vi "RTS Close TDMS.vi"(7 "RTS Config Setup Input":T2, 8 "Error In":errorcluster, 10 "Tree Selection":T1, 11 "TDMS Data Save in":T11) -> (0 "Error Out":errorcluster, 3 "RTS Config Setup Output":T2)   [LabVIEW 2016]
uses:
  Type Definitions/RTS TDMS Filename Locations.ctl
  Type Definitions/RTS Wago Config.ctl
  Type Definitions/RTS APLUS Config.ctl
  Type Definitions/RTS Yokogawa MX Config.ctl
  Type Definitions/RTS Replay Server Control.ctl
  Type Definitions/RTS Server Configuration.ctl
  Type Definitions/RTS Configuration Setup.ctl
  Type Definitions/RTS Station Settions TCP Comms.ctl
  Type Definitions/RTS Chamber Save Status.ctl
  Type Definitions/RTS Room Selector.ctl
  Type Definitions/RTS Test Pattern.ctl
  Type Definitions/RTS Save References.ctl
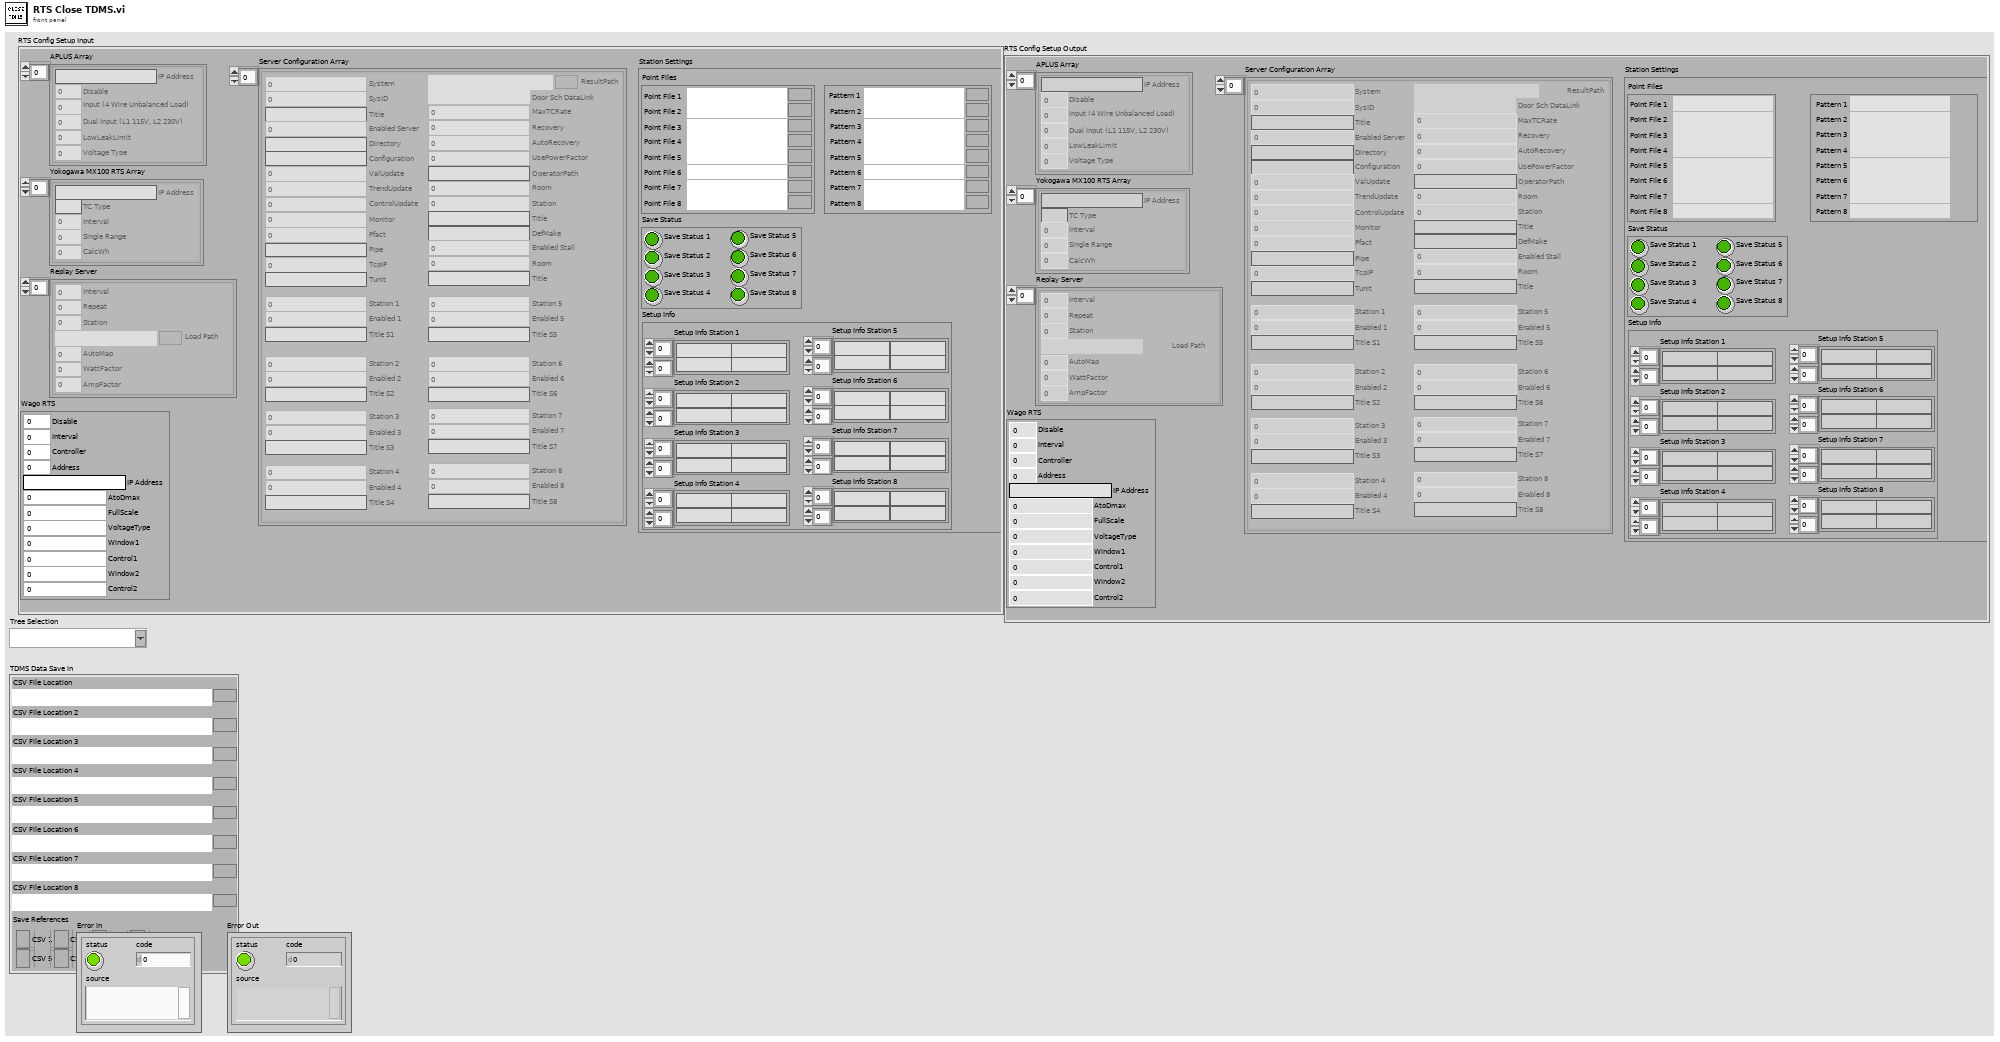
[diagram p1: front panel]
types:
  T1 = typedef "RTS Room Selector.ctl" = string
  T2 = typedef "RTS Configuration Setup.ctl" = cluster{"Wago RTS":T3, "APLUS Array":T4[], "Yokogawa MX100 RTS Array":T5[], "Replay Server":T6[], "Server Configuration Array":T7[], "Station Settings":T8}
  T3 = typedef "RTS Wago Config.ctl" = cluster{"Disable":u16, "Interval":u16, "Controller":u16, "Address":u16, "IP Address":string, "AtoDmax":u16, "FullScale":u16, "VoltageType":u16, "Window1":u16, "Control1":u16, "Window2":u16, "Control2":u16}
  T4 = typedef "RTS APLUS Config.ctl" = cluster{"Disable":u16, "IP Address":string, "Input (4 Wire Unbalanced Load)":u16, "Dual Input (L1 115V, L2 230V)":u16, "LowLeakLimit":dbl, "Voltage Type":u16}
  T5 = typedef "RTS Yokogawa MX Config.ctl" = cluster{"IP Address":string, "TC Type":string, "Interval":u16, "Single Range":u16, "CalcWh":u16}
  T6 = typedef "RTS Replay Server Control.ctl" = cluster{"Interval":i16, "Repeat":u16, "Station":u16, "Load Path":path, "AutoMap":u16, "WattFactor":dbl, "AmpFactor":dbl}
  T7 = typedef "RTS Server Configuration.ctl" = cluster{"System":u16, "SysID":u16, "Title":string, "Enabled Server":u16, "Directory":string, "Configuration":string, "ValUpdate":u16, "TrendUpdate":u16, "ControlUpdate":u16, "Monitor":u16, "Pfact":u16, "Pipe":string, "TcpIP":u16, "Tunit":string, "ResultPath":path, "Door Sch DataLink":path, "MaxTCRate":u16, "Recovery":u16, "AutoRecovery":u16, "UsePowerFactor":u16, "OperatorPath":string, "Room":u16, "Station":u16, "Title":string, "DefMake":string, "Enabled Stall":u16, "Room":u16, "Title":string, "Station 1":u16, "Enabled 1":u16, "Station 2":u16, "Enabled 2":u16, "Station 3":u16, "Enabled 3":u16, "Station 4":u16, "Enabled 4":u16, "Station 5":u16, "Enabled 5":u16, "Station 6":u16, "Enabled 6":u16, "Station 7":u16, "Enabled 7":u16, "Station 8":u16, "Enabled 8":u16, "Title S1":string, "Title S2":string, "Title S3":string, "Title S5":string, "Title S6":string, "Title S7":string, "Title S8":string, "Title S4":string}
  T8 = typedef "RTS Station Settions TCP Comms.ctl" = cluster{"Point Files":cluster{"Point File 1":path, "Point File 2":path, "Point File 3":path, "Point File 4":path, "Point File 5":path, "Point File 6":path, "Point File 7":path, "Point File 8":path}, "Save Status":T9, "Setup Info":cluster{"Setup Info Station 1":string[][], "Setup Info Station 2":string[][], "Setup Info Station 3":string[][], "Setup Info Station 4":string[][], "Setup Info Station 5":string[][], "Setup Info Station 6":string[][], "Setup Info Station 7":string[][], "Setup Info Station 8":string[][]}, "Chamber Test Pattern":T10}
  T9 = typedef "RTS Chamber Save Status.ctl" = cluster{"Save Status 1":bool, "Save Status 2":bool, "Save Status 3":bool, "Save Status 4":bool, "Save Status 5":bool, "Save Status 6":bool, "Save Status 7":bool, "Save Status 8":bool}
  T10 = typedef "RTS Test Pattern.ctl" = cluster{" Pattern 1":path, "Pattern 2":path, "Pattern 3":path, "Pattern 4":path, "Pattern 5":path, "Pattern 6":path, "Pattern 7":path, "Pattern 8":path}
  T11 = typedef "RTS TDMS Filename Locations.ctl" = cluster{"CSV File Location":path, "CSV File Location 2":path, "CSV File Location 3":path, "CSV File Location 4":path, "CSV File Location 5":path, "CSV File Location 6":path, "CSV File Location 7":path, "CSV File Location 8":path, "Save References":T12}
  T12 = typedef "RTS Save References.ctl" = cluster{"CSV 1":refnum<file>, "CSV 2":refnum<file>, "CSV 3":refnum<file>, "CSV 4":refnum<file>, "CSV 5":refnum<file>, "CSV 6":refnum<file>, "CSV 7":refnum<file>, "CSV 8":refnum<file>}
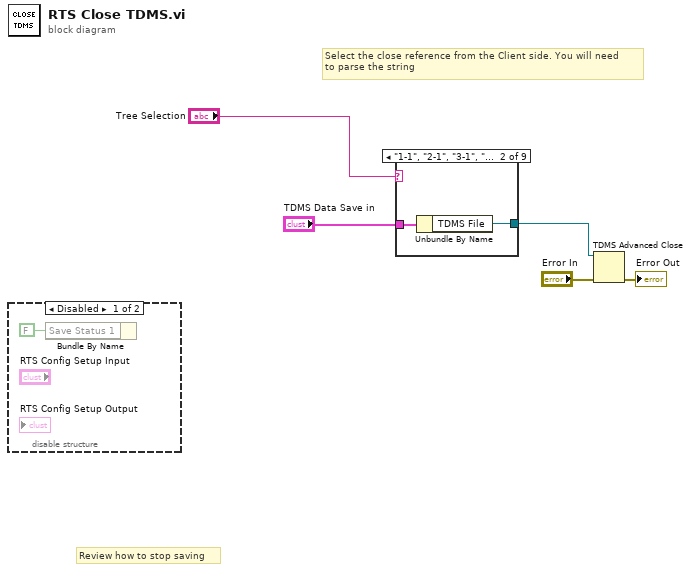
[diagram p0: block diagram]
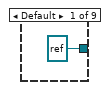
[diagram p3: hidden frame]
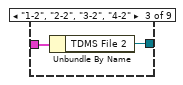
[diagram p4: hidden frame]
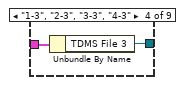
[diagram p5: hidden frame]
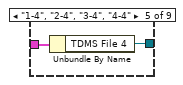
[diagram p6: hidden frame]
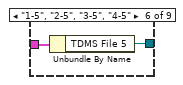
[diagram p7: hidden frame]
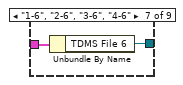
[diagram p8: hidden frame]
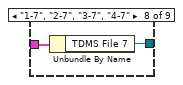
[diagram p9: hidden frame]
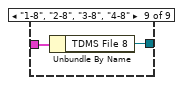
[diagram p10: hidden frame]
diagram:
  # "Review how to stop saving"
  # "Select the close reference from the Client side. You will need\nto parse the string"
  n1 = disable-structure shown="Disabled" {
    frame Disabled {
      n2 = Bundle By Name("Save Status 1"=FALSE ("Station Saving 8")) -> ()  [unwired: 1 in, 1 out]
    }
    frame Enabled {
    }
  }
  n3 = case shown="\"1-1\", \"2-1\", \"3-1\", \"4-1\"" "Tree Selection" {
    tunnel: "TDMS Data Save in" -> [_ w9 w11 w13 w15 w17 w19 w21 w23]
    tunnel: [refnum<k34> refnum ("TDMS File 8") w8 w10 w12 w14 w16 w18 w20 w22] -> w2
    frame Default {
    }
    frame "1-1", "2-1", "3-1", "4-1" {
      n4 = Unbundle By Name(w9) -> ("TDMS File"=w8:refnum<k34>)
    }
    frame "1-2", "2-2", "3-2", "4-2" {
      n5 = Unbundle By Name(w11) -> ("TDMS File 2"=w10:refnum<k34>)
    }
    frame "1-3", "2-3", "3-3", "4-3" {
      n6 = Unbundle By Name(w13) -> ("TDMS File 3"=w12:refnum<k34>)
    }
    frame "1-4", "2-4", "3-4", "4-4" {
      n7 = Unbundle By Name(w15) -> ("TDMS File 4"=w14:refnum<k34>)
    }
    frame "1-5", "2-5", "3-5", "4-5" {
      n8 = Unbundle By Name(w17) -> ("TDMS File 5"=w16:refnum<k34>)
    }
    frame "1-6", "2-6", "3-6", "4-6" {
      n9 = Unbundle By Name(w19) -> ("TDMS File 6"=w18:refnum<k34>)
    }
    frame "1-7", "2-7", "3-7", "4-7" {
      n10 = Unbundle By Name(w21) -> ("TDMS File 7"=w20:refnum<k34>)
    }
    frame "1-8", "2-8", "3-8", "4-8" {
      n11 = Unbundle By Name(w23) -> ("TDMS File 8"=w22:refnum<k34>)
    }
  }
  n12 = TDMS Advanced Close(8:"Error In", 11:w2) -> (0:→"Error Out":errorcluster)  [unwired: 2 in, 1 out]
